vi "Replace Stats Page.vi"(0 "Filepath":path, 7 "Data":string[][](array[string]), 11 "Error In":errorcluster) -> (15 "Error Out":errorcluster)   [LabVIEW 2013]
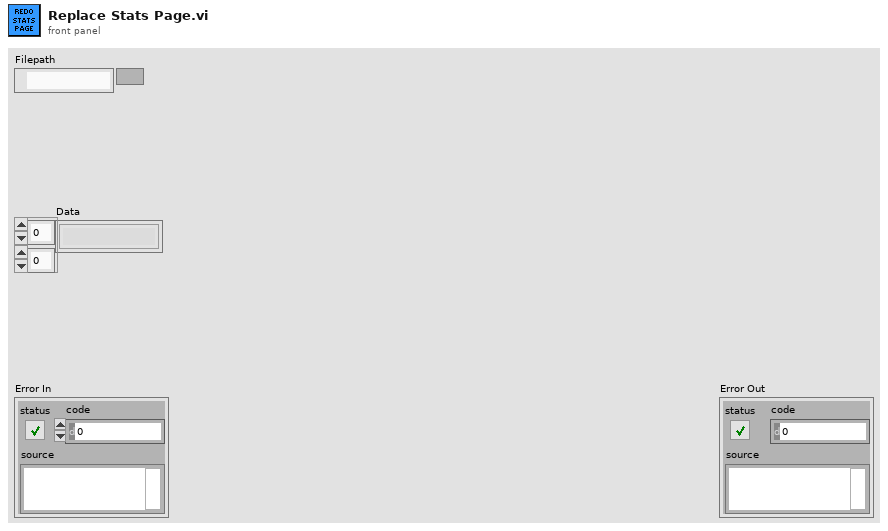
[diagram p1: front panel]
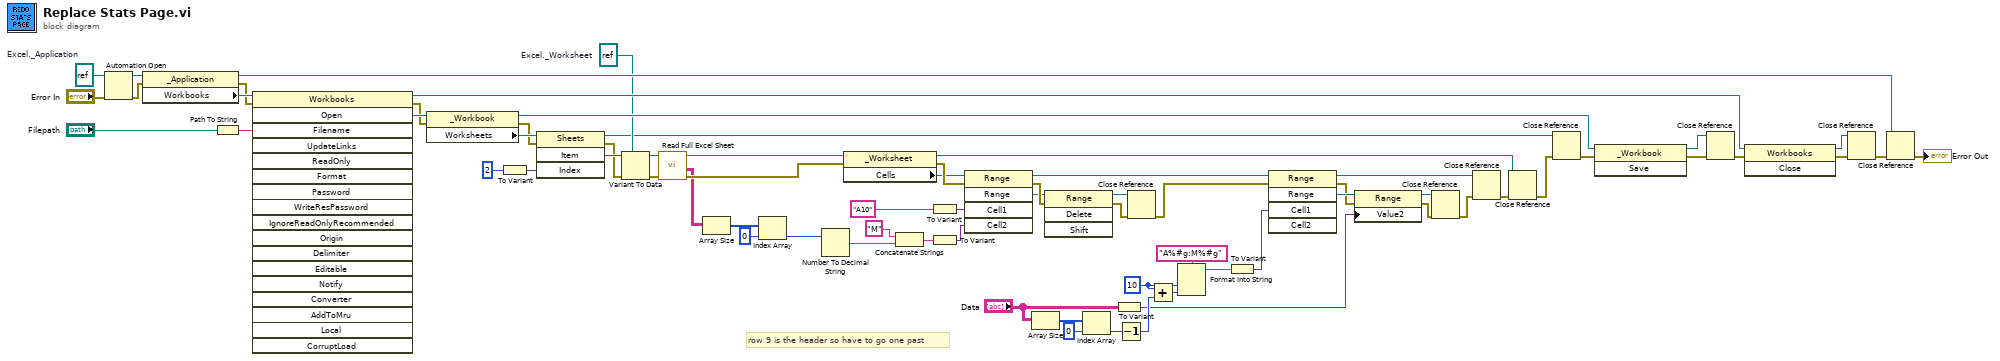
[diagram p0: block diagram]
diagram:
  w8 = 10 ("index")
  w35 = refnum<k7> refnum  # Excel._Worksheet
  w68 = refnum<k7> refnum  # Excel._Application
  # "row 9 is the header so have to go one past"
  n1 = Automation Open(error in (no error)="Error In", Automation Refnum=w68) -> (Automation Refnum=w69:refnum<k7>, error out=w70:errorcluster)  [unwired: 2 in]
  n2 = property class="_Application"(reference=w69, error in=w70) -> (reference out=w61:refnum<k7>, error out=w62:errorcluster, "Workbooks"=w71:refnum<k7>)
  n3 = Path To String(path="Filepath") -> (string=w58:string)
  n4 = invoke class="Workbooks" method="Open"(reference=w71, error in=w62, "Filename"=w58) -> (reference out=w65:refnum<k7>, error out=w60:errorcluster, "Open"=w67:refnum<k7>)  [unwired: 15 in, 15 out]
  n5 = property class="_Workbook"(reference=w67, error in=w60) -> (reference out=w54:refnum<k7>, error out=w29:errorcluster, "Worksheets"=w30:refnum<k7>)
  n6 = To Variant(anything=2) -> (Variant=w36:variant)
  n7 = invoke class="Sheets" method="Item"(reference=w30, error in=w29, "Index"=w36) -> (reference out=w34:refnum<k7>, error out=w33:errorcluster, "Item"=w37:variant)  [unwired: 1 in, 1 out]
  n8 = Variant To Data(error in=w33, type=w35, Variant=w37) -> (data=w28:refnum<k7>, error out=w27:errorcluster)
  n9 = call "Read Full Excel Sheet.vi"("Error In"=w27, "Excel._Worksheet"=w28) -> ("Error Out"=w25:errorcluster, "Data"=w24:string[][], "Reference Out"=w26:refnum<k7>)  [unwired: 7 in]
  n10 = Array Size(array=w24) -> (size(s)=w23:i32[])
  n11 = Index Array(array=w23, index=0) -> (element=w21:i32)
  n12 = Number To Decimal String(number=w21) -> (decimal integer string=w31:string)  [unwired: 1 in]
  n13 = property class="_Worksheet"(reference=w26, error in=w25) -> (reference out=w39:refnum<k7>, error out=w43:errorcluster, "Cells"=w42:refnum<k7>)
  n14 = Concatenate Strings("M" ("ColumnIndex"), w31) -> (w49:string)
  n15 = To Variant(anything="A10" ("ColumnIndex")) -> (Variant=w41:variant)
  n16 = To Variant(anything=w49) -> (Variant=w45:variant)
  n17 = invoke class="Range" method="Range"(reference=w42, error in=w43, "Cell1"=w41, "Cell2"=w45) -> (reference out=w7:refnum<k7>, error out=w46:errorcluster, "Range"=w44:refnum<k7>)  [unwired: 1 in, 2 out]
  n18 = Array Size(array="Data") -> (size(s)=w15:i32[])
  n19 = invoke class="Range" method="Delete"(reference=w44, error in=w46) -> (reference out=w47:refnum<k7>, error out=w48:errorcluster)  [unwired: 2 in, 2 out]
  n20 = Index Array(array=w15, index=0) -> (element=w17:i32)
  n21 = To Variant(anything="Data") -> (Variant=w11:variant)
  n22 = Decrement(x=w17) -> (x-1=w18:i32)
  n23 = Close Reference(reference=w47, error in (no error)=w48) -> (error out=w6:errorcluster)
  n24 = Add(x=w8, y=w18) -> (x+y=w14:i32)
  n25 = Format Into String(format string="A%#g:M%#g", w8, w14) -> (resulting string=w12:string)  [unwired: 2 in, 1 out]
  n26 = To Variant(anything=w12) -> (Variant=w10:variant)
  n27 = invoke class="Range" method="Range"(reference=w7, error in=w6, "Cell1"=w10) -> (reference out=w5:refnum<k7>, error out=w4:errorcluster, "Range"=w13:refnum<k7>)  [unwired: 2 in, 2 out]
  n28 = property class="Range"(reference=w13, error in=w4, "Value2"=w11) -> (reference out=w2:refnum<k7>, error out=w3:errorcluster)
  n29 = Close Reference(reference=w2, error in (no error)=w3) -> (error out=w1:errorcluster)
  n30 = Close Reference(reference=w5, error in (no error)=w1) -> (error out=w38:errorcluster)
  n31 = Close Reference(reference=w39, error in (no error)=w38) -> (error out=w32:errorcluster)
  n32 = Close Reference(reference=w34, error in (no error)=w32) -> (error out=w59:errorcluster)
  n33 = invoke class="_Workbook" method="Save"(reference=w54, error in=w59) -> (reference out=w55:refnum<k7>, error out=w56:errorcluster)  [unwired: 1 in, 1 out]
  n34 = Close Reference(reference=w55, error in (no error)=w56) -> (error out=w57:errorcluster)
  n35 = invoke class="Workbooks" method="Close"(reference=w65, error in=w57) -> (reference out=w64:refnum<k7>, error out=w63:errorcluster)  [unwired: 1 in, 1 out]
  n36 = Close Reference(reference=w64, error in (no error)=w63) -> (error out=w66:errorcluster)
  n37 = Close Reference(reference=w61, error in (no error)=w66) -> (error out=→"Error Out":errorcluster)
